vi "End Str.vi"   [LabVIEW 2019, in "LabPack.lvlib" / "Reader.lvclass"]
doc: "Finishes decoding a string. This must be called after reading all of the data for the string; otherwise, an error will occur with any following Reader VIs."
uses:
  Reader.lvclass
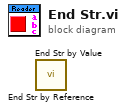
[diagram p0: block diagram]
diagram:
  n1 = call "End Str by Reference.vi"() -> ()  [unwired: 10 in, 2 out]
  n2 = call "End Str by Value.vi"() -> ()  [unwired: 10 in, 2 out]
